vi "CheckIfAborted.vi"(8 "error in":errorcluster, 11 "reference in":refnum<vi>) -> (0 "error out":errorcluster, 2 "Abort?":bool, 3 "reference out":refnum<vi>)   [LabVIEW 2020]
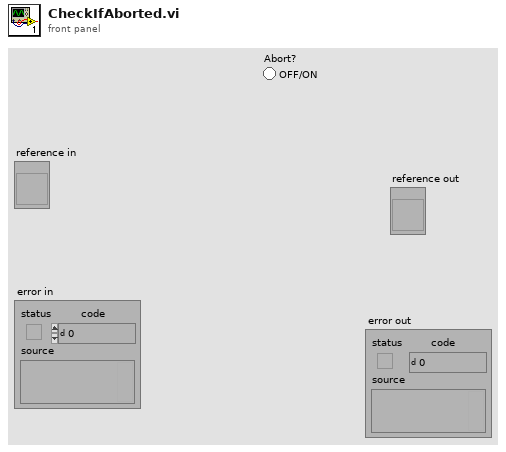
[diagram p1: front panel]
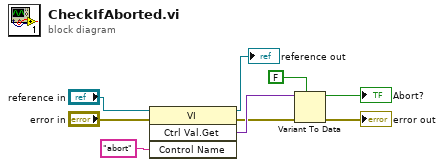
[diagram p0: block diagram]
diagram:
  n1 = invoke class="VI" method="Ctrl Val.Get"(reference="reference in", error in="error in", "Control Name"="abort") -> (reference out=→"reference out":refnum<vi>, error out=w3:errorcluster, "Get Control Value Variant"=w7:variant)  [unwired: 1 in, 1 out]
  n2 = Variant To Data(error in=w3, type=FALSE ("stop"), Variant=w7) -> (data=→"Abort?":bool, error out=→"error out":errorcluster)
